vi "Hot_wire_Calculator.vi"() -> ()   [LabVIEW 2010]
panel:
  out "Hot Wire Hot Resistance":dbl format="%.2f"
  out "Resistance that should be set":dbl format="%.2f"
  out "Hot Wire Cold Resistance":dbl format="%.2f"
  in  "Overheat Ratio":dbl=0.75 min=0.0 max=1.0 step=0.05 format="%.2f"
  in  "Resistance with Hot Wire Probe":dbl format="%.2f"
  in  "Resistance with Shorting Probe":dbl format="%.2f"
  # "Input Information"
  # "Rhot-Rcold\n   Rcold"
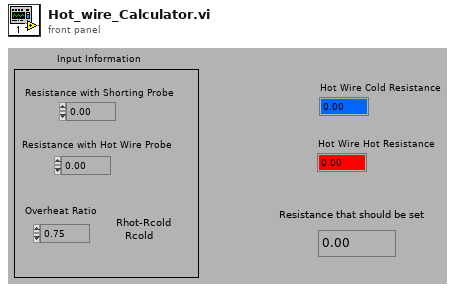
[diagram p1: front panel]
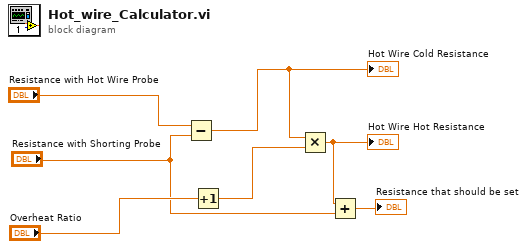
[diagram p0: block diagram]
diagram:
  n1 = Subtract(x="Resistance with Hot Wire Probe", y="Resistance with Shorting Probe") -> (x-y=w6:dbl)
  "Hot Wire Cold Resistance" <- w6
  n2 = Increment(x="Overheat Ratio") -> (x+1=w4:dbl)
  n3 = Multiply(x=w6, y=w4) -> (x*y=w3:dbl)
  "Hot Wire Hot Resistance" <- w3
  n4 = Add(x=w3, y="Resistance with Shorting Probe") -> (x+y=→"Resistance that should be set":dbl)
